vi "Abort All.vi"(11 "Test Case In":refnum<class "Tests Event MessengerM.lvclass">) -> (0 "error out":errorcluster, 3 "Test Case Out":refnum<class "Tests Event MessengerM.lvclass">)   [LabVIEW 2020, in "Tests Event MessengerM.lvclass"]
uses:
  Tests Event MessengerM.lvclass
  C:/Program Files/National Instruments/LabVIEW 2026/vi.lib/Astemes/LUnit/Test Case.lvclass
  <vilib>/Astemes/LUnit/Test Case.lvclass/Test Case.ctl
  Tests Event MessengerM.lvclass/Tests Event MessengerM.ctl
  <vilib>/Astemes/LUnit/Test Case.lvclass
  71af0f09-12c7-4dfe-8abc-e79a1d10b62a.vi
  2885cf67-225c-494c-b9be-b79676d4dd65.vi
  4deba37e-ab4d-45f5-82a8-5b4237af5526.vi
  9d005ed5-dfb0-446f-bee6-5e90b4191148.vi
panel:
  out "cmd 2":string
  out "cmd":string
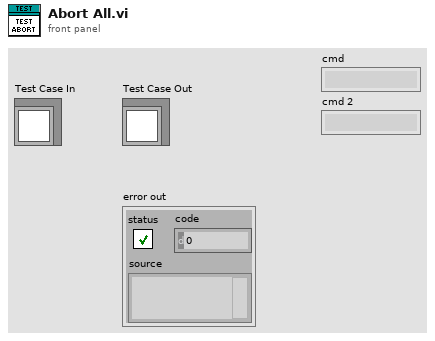
[diagram p1: front panel]
types:
  T1 = typedef "Event MessengerM-c(str,var).lvlib/))Channel.ctl" = refnum<queue>
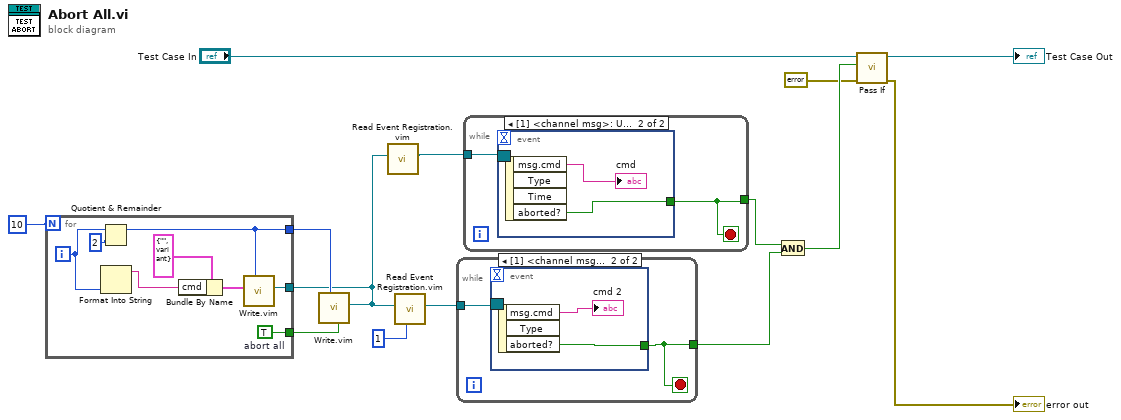
[diagram p0: block diagram]
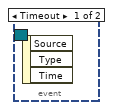
[diagram p2: hidden frame]
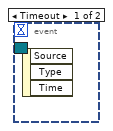
[diagram p3: hidden frame]
diagram:
  n1 = for {
    N: 10 -> [_]
    tunnel: [w16] -> w5
    tunnel: [w15] -> w3
    tunnel: [w18] -> w6
    i -> [w20]
    w18 = TRUE  # abort all
    n2 = Quotient & Remainder(x=w20, y=2) -> (x-y*floor(x/y)=w16:i32)  [unwired: 1 out]
    n3 = Format Into String(w20) -> (resulting string=w19:string)  [unwired: 3 in, 1 out]
    n4 = Bundle By Name(cluster=cluster{"cmd":string, "data":variant} {"cmd"="", "data"=variant} ("element"), "cmd"=w19) -> (w17:cluster{"cmd":string, "data":variant})
    n5 = call "Write.vim"("subchannel"=w16, "element"=w17) -> ("channel"=w15:T1)  [unwired: 8 in, 1 out]
  }
  n6 = call "Write.vim"("channel"=w3, "abort all (F)"=w6, "subchannel"=w5) -> ()  [unwired: 8 in, 1 out]
  n7 = call "Read Event Registration.vim"("channel"=w3) -> ("event registration refnum"=w4:refnum<event-registration>)  [unwired: 10 in]
  n8 = call "Read Event Registration.vim"("subchannel"=1 ("subchannel (0)"), "channel"=w3) -> ("event registration refnum"=w2:refnum<event-registration>)  [unwired: 9 in]
  n9 = while {
    tunnel: [w24] -> w9
    tunnel: w2 -> [w23]
    stop <- w24 stop-if-true
    n10 = event shown="[1] <channel msg>: User Event" {
      selector: w23 -> [_ _]
      dyn-events: _ -> [_ _]
      timeout: _ -> [_ _]
      tunnel: [_ w25] -> w24
      event Timeout {
        n11 = event-data() -> ()  [unwired: 1 in, 3 out]
      }
      event User Event {
        n12 = event-data() -> ("msg.cmd"=→"cmd 2":string, "aborted?"=w25:bool)  [unwired: 1 in, 1 out]
      }
    }
  }
  n13 = while {
    tunnel: [w28] -> w8
    tunnel: w4 -> [w27]
    stop <- w28 stop-if-true
    n14 = event shown="[1] <channel msg>: User Event" {
      selector: w27 -> [_ _]
      dyn-events: _ -> [_ _]
      timeout: _ -> [_ _]
      tunnel: [_ w30] -> w28
      event Timeout {
        n15 = event-data() -> ()  [unwired: 1 in, 3 out]
      }
      event User Event {
        n16 = event-data() -> ("msg.cmd"=→"cmd":string, "aborted?"=w30:bool)  [unwired: 1 in, 2 out]
      }
    }
  }
  n17 = And(x=w8, y=w9) -> (x .and. y?=w10:bool)
  n18 = call <vilib>:"Pass If.vi"("error in (no error)"=errorcluster {"status"=FALSE, "code"=0, "source"=""}, "Pass?"=w10, "LUnit Test Case In"="Test Case In") -> ("error out"=→"error out":errorcluster, "LUnit Test Case Out"=→"Test Case Out":refnum<class "Tests Event MessengerM.lvclass">)  [unwired: 7 in]
